vi "cleanWaypoints.vi"(8 "error in (no error)":errorcluster, 10 "Waypoint Queue":refnum<queue>, 11 "Old Waypoints":refnum<class "Waypoint.lvclass">[](array[class])) -> (0 "error out":errorcluster, 2 "Done?":bool, 3 "Old Waypoints (updated)":refnum<class "Waypoint.lvclass">[](array[class]))   [LabVIEW 2013]
doc: "When the next waypoints has been marked done, remove it from the queue and add it to the waypoint history array"
uses:
  Logic/Classes/Waypoint/Waypoint.lvclass
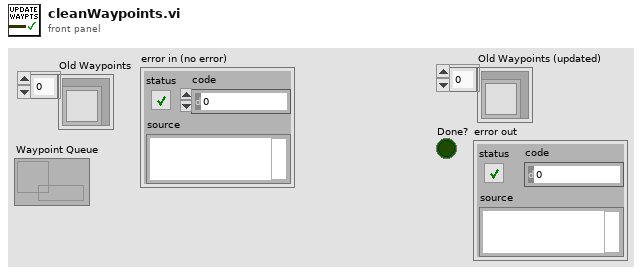
[diagram p1: front panel]
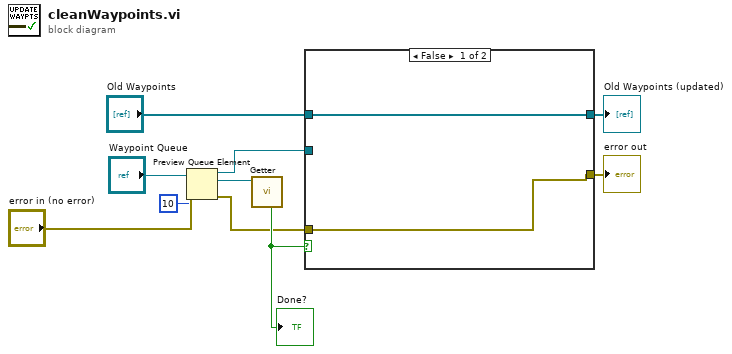
[diagram p0: block diagram]
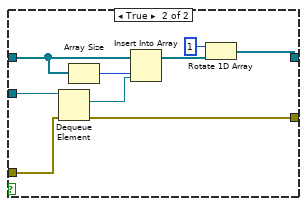
[diagram p2: hidden frame]
diagram:
  n1 = Preview Queue Element(queue="Waypoint Queue", timeout in ms (-1)=10, error in (no error)="error in (no error)") -> (queue out=w7:refnum<queue>, element=w9:refnum<class "Waypoint.lvclass">, error out=w3:errorcluster)  [unwired: 1 out]
  n2 = call "Getter.vi"("Waypoint In"=w9) -> ("Done?"=w8:bool)  [unwired: 6 in, 4 out]
  "Done?" <- w8
  n3 = case shown="False" w8 {
    tunnel: w7 -> [_ w21]
    tunnel: "Old Waypoints" -> [w12 w19]
    tunnel: [w12 w15] -> w5
    tunnel: w3 -> [w11 w14]
    tunnel: [w11 w13] -> w2
    frame False {
    }
    frame True {
      n4 = Dequeue Element(queue=w21, error in (no error)=w14) -> (element=w20:refnum<class "Waypoint.lvclass">, error out=w13:errorcluster)  [unwired: 1 in, 2 out]
      n5 = Array Size(array=w19) -> (size(s)=w18:i32)
      n6 = Insert Into Array(array=w19, index=w18, new element=w20) -> (w17:refnum<class "Waypoint.lvclass">[])
      n7 = Rotate 1D Array(1:w17, 2:1 ("n")) -> (0:w15:refnum<class "Waypoint.lvclass">[])
    }
  }
  "Old Waypoints (updated)" <- w5
  "error out" <- w2
